vi "Example_CT.vi"() -> ()   [LabVIEW 2024]
uses:
  Update Method.ctl
  Cyclic Table.lvclass
panel:
  in  "Update Method (FIFO)":T1=enum."New Top"
  in  "Rows":i32=10
  in  "stop":bool
  in  "Freeze Display":bool
  out "Table Control":string[][](table)
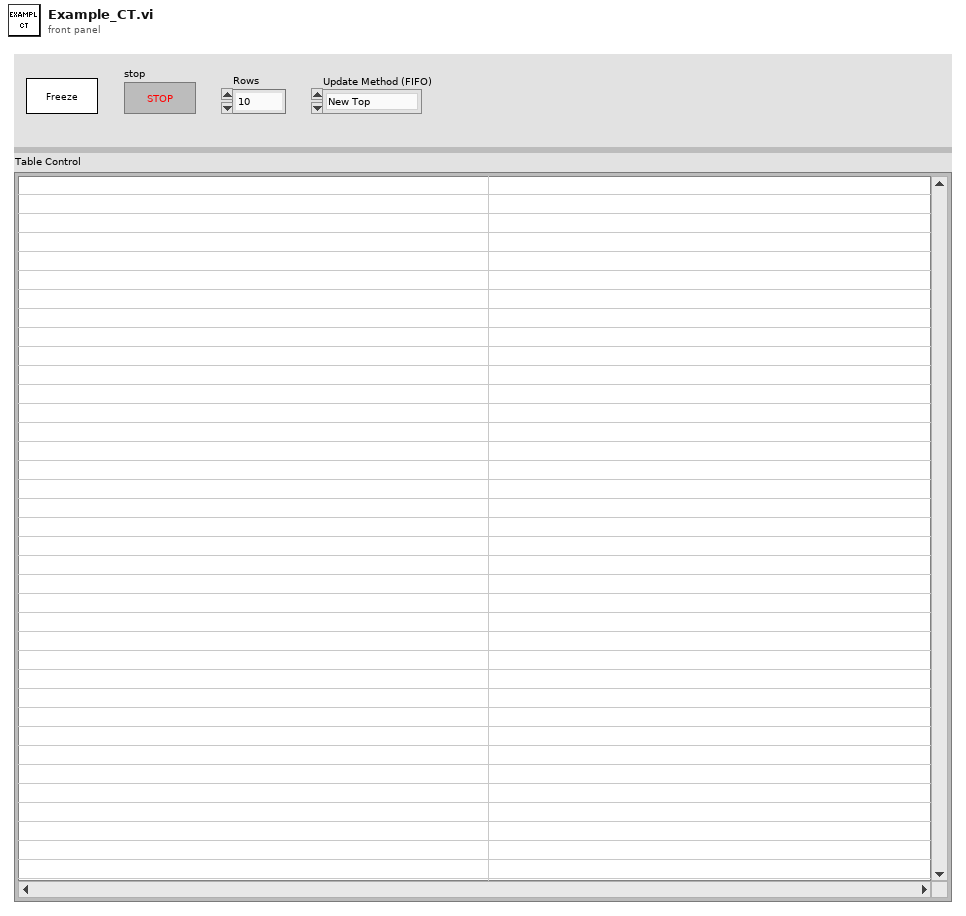
[diagram p1: front panel]
types:
  T1 = typedef "Cyclic Table.lvclass/Update Method.ctl" = enum16{"Cyclic", "Old Top", "New Top"}
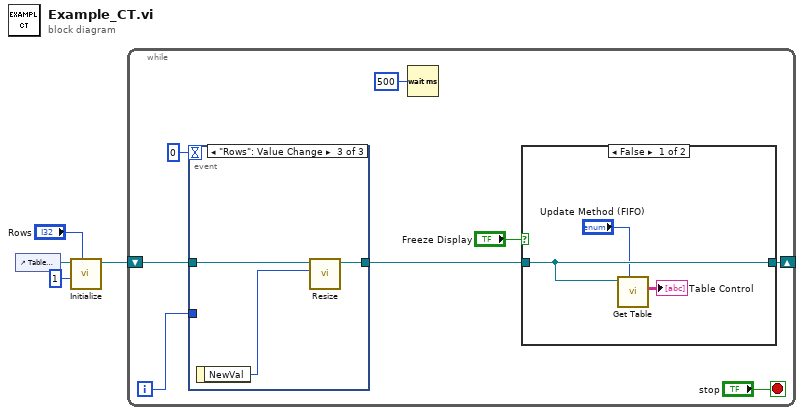
[diagram p0: block diagram]
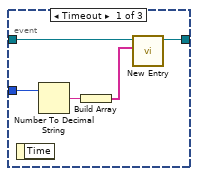
[diagram p2: hidden frame]
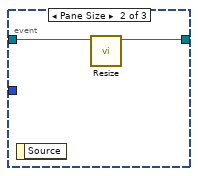
[diagram p3: hidden frame]
diagram:
  n1 = control-ref of="Table Control"() -> (w4:refnum<vi>)
  n2 = call "Initialize.vi"("rows (auto from ref)"="Rows", "# columns"=1, "Table"=w4) -> ("Cyclic Table"=w3:refnum<class "Cyclic Table.lvclass">)  [unwired: 7 in, 1 out]
  n3 = while {
    shift-right: [w7] -> _
    shift-left: w3 -> [w10]
    i -> [w9]
    stop <- "stop" stop-if-true
    n4 = event shown="[2] \"Rows\": Value Change" {
      selector: _ -> [_ _ _]
      dyn-events: _ -> [_ _ _]
      timeout: 0 -> [_ _ _]
      tunnel: w10 -> [w17 w19 w22]
      tunnel: w9 -> [w16 _ _]
      tunnel: [w13 w18 w21] -> w8
      event Timeout {
        n5 = event-data() -> ()  [unwired: 1 in, 1 out]
        n6 = Number To Decimal String(number=w16) -> (decimal integer string=w15:string)  [unwired: 1 in]
        n7 = Build Array(w15) -> (w14:string[])
        n8 = call "New Entry.vi"("New Entry"=w14, "Cyclic Table in"=w17) -> ("Cyclic Table out"=w13:refnum<class "Cyclic Table.lvclass">)  [unwired: 9 in]
      }
      event Pane Size {
        n9 = event-data() -> ()  [unwired: 1 in, 1 out]
        n10 = call "Resize.vi"("Cyclic Table in"=w19) -> ("Cyclic Table out"=w18:refnum<class "Cyclic Table.lvclass">)  [unwired: 10 in]
      }
      event "Rows": Value Change {
        n11 = event-data() -> ("NewVal"=w20:i32)  [unwired: 1 in]
        n12 = call "Resize.vi"("Number of Rows (auto from ref)"=w20, "Cyclic Table in"=w22) -> ("Cyclic Table out"=w21:refnum<class "Cyclic Table.lvclass">)  [unwired: 9 in]
      }
    }
    n13 = Wait (ms)(milliseconds to wait=u32 500) -> ()  [unwired: 1 out]
    n14 = case shown="False" "Freeze Display" {
      tunnel: w8 -> [w25 w26]
      tunnel: [w25 w26] -> w7
      frame False {
        n15 = call "Get Table.vi"("Update Method (New Top)"="Update Method (FIFO)", "Cyclic Table in"=w25) -> ("Table Data (sorted by time)"=→"Table Control":string[][])  [unwired: 9 in]
      }
      frame True {
      }
    }
  }
